vi "Prompt for Step--Init UI.vi"(8 "error in (no error)":errorcluster, 10 "Control Ref Map":map{string, refnum<vi>}(c390), 11 "Window Action in":refnum<class "Window Action.lvclass">) -> (0 "error out":errorcluster, 3 "Window Action out":refnum<class "Window Action.lvclass">)   [LabVIEW 2020, in "MacroAssert.lvlib" / "Window Action.lvclass"]
doc: "Initializes the user interface within the \"Prompt for Step\" VI."
uses:
  Window Action.lvclass
  d8e374d7-7127-4221-b5e7-bd2a4e3622c5.vi
  Support/Get Control Reference by Label (1D STR).vi
  <vilib>/Utility/error.llb/Error Cluster From Error Code.vi
  Action Step/Action Step.lvclass
  MacroAssert.lvlib
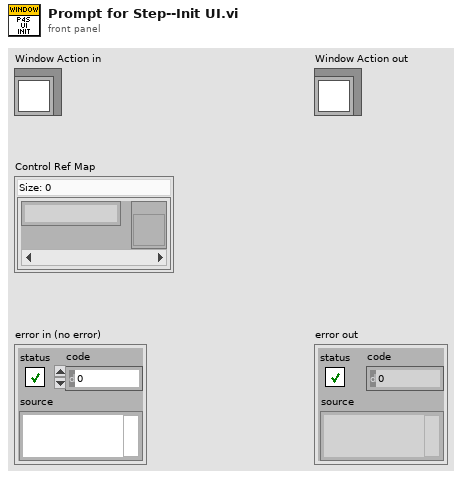
[diagram p1: front panel]
types:
  T1 = typedef "MacroAssert.lvlib/Window Action.lvclass/Window Action Type.ctl" = enum16{"Maximize Window", "Restore Window", "Minimize Window", "Close Window", "Bring Window to Front", "Send Window to Back"}
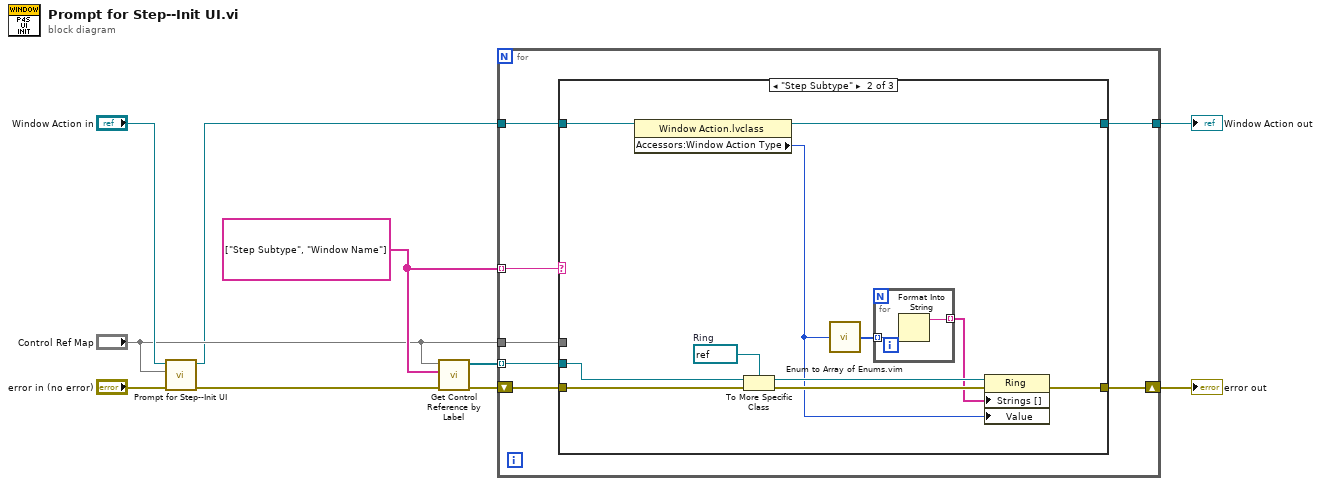
[diagram p0: block diagram]
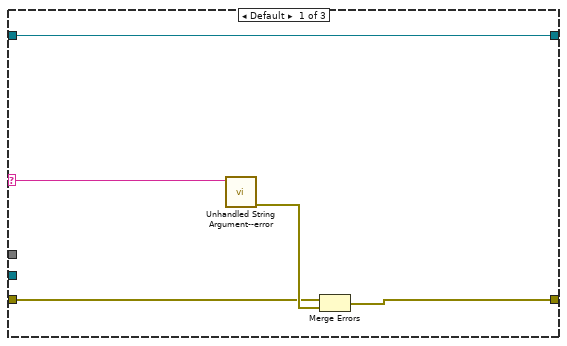
[diagram p2: hidden frame]
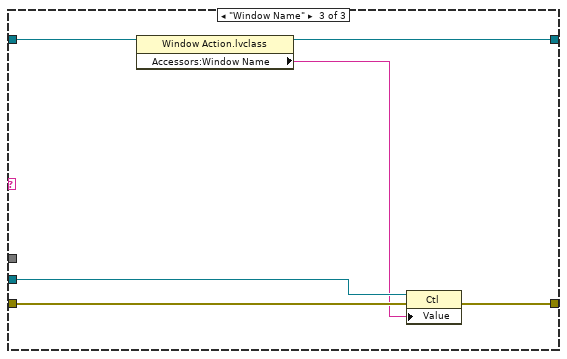
[diagram p3: hidden frame]
diagram:
  w9 = string[] ["Step Subtype", "Window Name"]
  n1 = call-parent "Prompt for Step--Init UI.vi"("error in (no error)"="error in (no error)", "Control Ref Map"="Control Ref Map", "Step in"="Window Action in") -> ("error out"=w4:errorcluster, "Step out"=w1:refnum<class "Window Action.lvclass">)  [unwired: 7 in]
  n2 = call-poly "Get Control Reference by Label.vi"("error in (no error)"=w4, "Control Names"=w9, "Control Ref Map"="Control Ref Map") -> ("error out"=w10:errorcluster, "Control Refs"=w8:refnum<vi>[])  [unwired: 6 in, 1 out]
  n3 = for {
    tunnel: w1 -> [w15]
    tunnel: [w13] -> w5
    tunnel: w9 -> [w16] mode=indexing
    tunnel: w8 -> [w14] mode=indexing
    shift-right: [w12] -> w7
    shift-left: w10 -> [w17]
    tunnel: "Control Ref Map" -> [w11]
    n4 = case shown="\"Step Subtype\"" w16 {
      selector: w16 -> [w19 _ _]
      tunnel: w17 -> [w20 w25 w38]
      tunnel: w15 -> [w22 w27 w41]
      tunnel: w14 -> [_ w24 w39]
      tunnel: [w22 w23 w40] -> w13
      tunnel: [w18 w26 w36] -> w12
      tunnel: w11 -> [_ _ _]
      frame Default {
        n5 = call "Unhandled String Argument--error.vi"("Argument"=w19) -> ("error out"=w21:errorcluster)  [unwired: 10 in]
        n6 = Merge Errors(w20, w21) -> (w18:errorcluster)
      }
      frame "Step Subtype" {
        w30 = refnum<vi> refnum  # Ring
        n7 = property class="Window Action.lvclass"(reference=w27) -> (reference out=w23:refnum<class "Window Action.lvclass">, "Accessors:Window Action Type"=w29:T1)  [unwired: 1 in, 1 out]
        n8 = To More Specific Class(target class=w30, reference=w24, error in=w25) -> (specific class reference=w33:refnum<vi>, error out=w31:errorcluster)
        n9 = call "Enum to Array of Enums.vim"("enum"=w29) -> ("array of enums"=w32:T1[])
        n10 = for {
          tunnel: w32 -> [w35] mode=indexing
          tunnel: [w34] -> w28 mode=indexing
          n11 = Format Into String(w35) -> (resulting string=w34:string)  [unwired: 3 in, 1 out]
        }
        n12 = property class="Ring"(reference=w33, error in=w31, "Strings []"=w28, "Value"=w29) -> (error out=w26:errorcluster)  [unwired: 1 out]
      }
      frame "Window Name" {
        n13 = property class="Window Action.lvclass"(reference=w41) -> (reference out=w40:refnum<class "Window Action.lvclass">, "Accessors:Window Name"=w37:string)  [unwired: 1 in, 1 out]
        n14 = property class="Ctl"(reference=w39, error in=w38, "Value"=w37) -> (error out=w36:errorcluster)  [unwired: 1 out]
      }
    }
  }
  "error out" <- w7
  "Window Action out" <- w5
